vi "Evaluate Alarms.vi"(0 "In Test":bool, 1 "Controller":T1, 2 "Alarm Config":T3, 3 "Data":dbl[](array[numeric]), 4 "Pumps Present":bool[](array[boolean])=[FALSE, FALSE, FALSE, FALSE, FALSE, FALSE], 5 "Trip Counter":i32[](array[numeric]), 6 "Previous Times":u32[](array[numeric]), 7 "Manual CMDs":dbl[](array[numeric]), 9 "Prev ON Times":u32[](array[numeric])) -> (20 "Trip Counter OUT":i32[](array[numeric]), 21 "Previous Times OUT":u32[](array[numeric]), 22 "Alarm Tripped":bool, 24 "Prev ON Times OUT":u32[](array[numeric]), 25 "Alarm Message 1":string, 26 "Alarm Message 2":string)   [LabVIEW 2019]
uses:
  Controls/Alarm Config.ctl
  Controls/Alarm Definition.ctl
  Controls/Alarm Profile Config.ctl
  Controls/Controller Config.ctl
  Type Defs/Controller Names.ctl
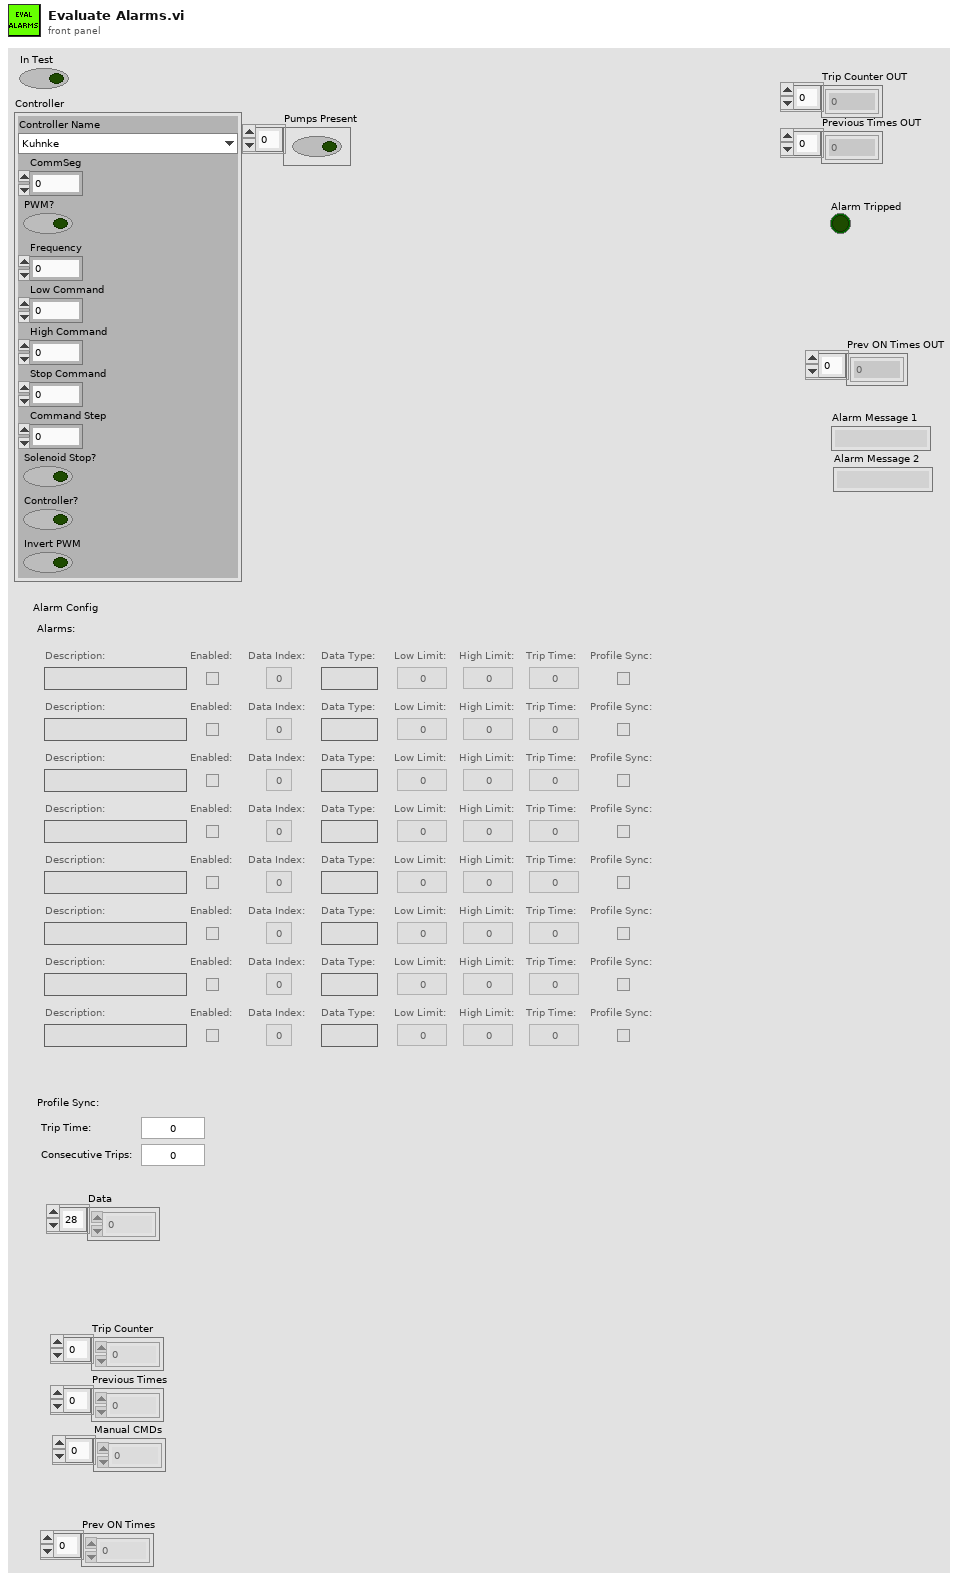
[diagram p1: front panel]
types:
  T1 = typedef "Controller Config.ctl" = cluster{"Controller Name":T2, "CommSeg":i32, "PWM?":bool, "Frequency":i32, "Low Command":dbl, "High Command":dbl, "Stop Command":dbl, "Command Step":dbl, "Solenoid Stop?":bool, "Controller?":bool, "Invert PWM":bool}
  T2 = typedef "Controller Names.ctl" = enum16{"Kuhnke", "Helbako BLDC", "Conti", "Hella BLDC OL PWM", "Hella BLDC Turbine OL PWM", "Hella BLDC Pressure", "Helbako (old)", "TI PWM", "PSA", "Hella Gas", "Hella Diesel", "8 Comm", "10 Comm", "8 Comm Hella", "10 Comm Hella", "8 Comm Omron", "10 Comm Omron", "8 Comm Nissan", "10 Comm Nissan"}
  T3 = typedef "Alarm Config.ctl" = cluster{"Alarms:":T4[], "Profile Sync:":T5}
  T4 = typedef "Alarm Definition.ctl" = cluster{"Description:":string, "Enabled:":bool, "Data Index:":i32, "Data Type:":string, "Low Limit:":dbl, "High Limit:":dbl, "Trip Time:":u32, "Profile Sync:":bool}
  T5 = typedef "Alarm Profile Config.ctl" = cluster{"Trip Time:":u32, "Consecutive Trips:":i32}
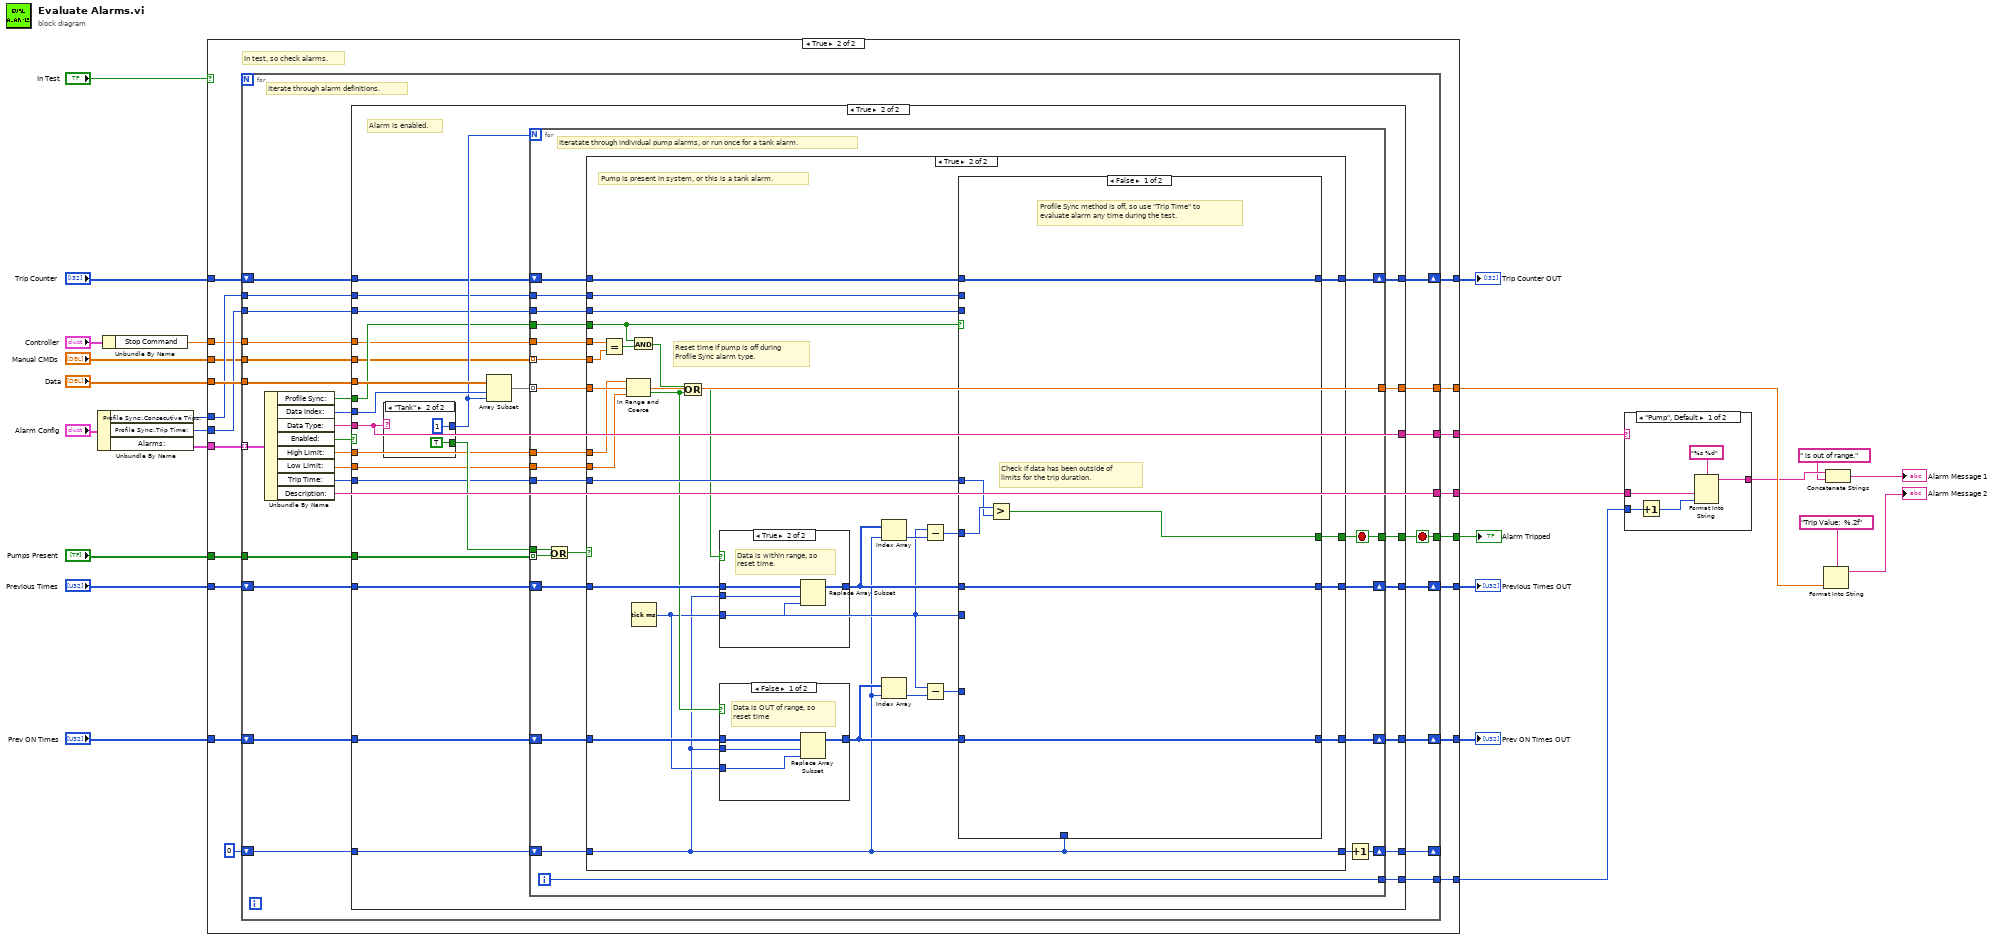
[diagram p0: block diagram]
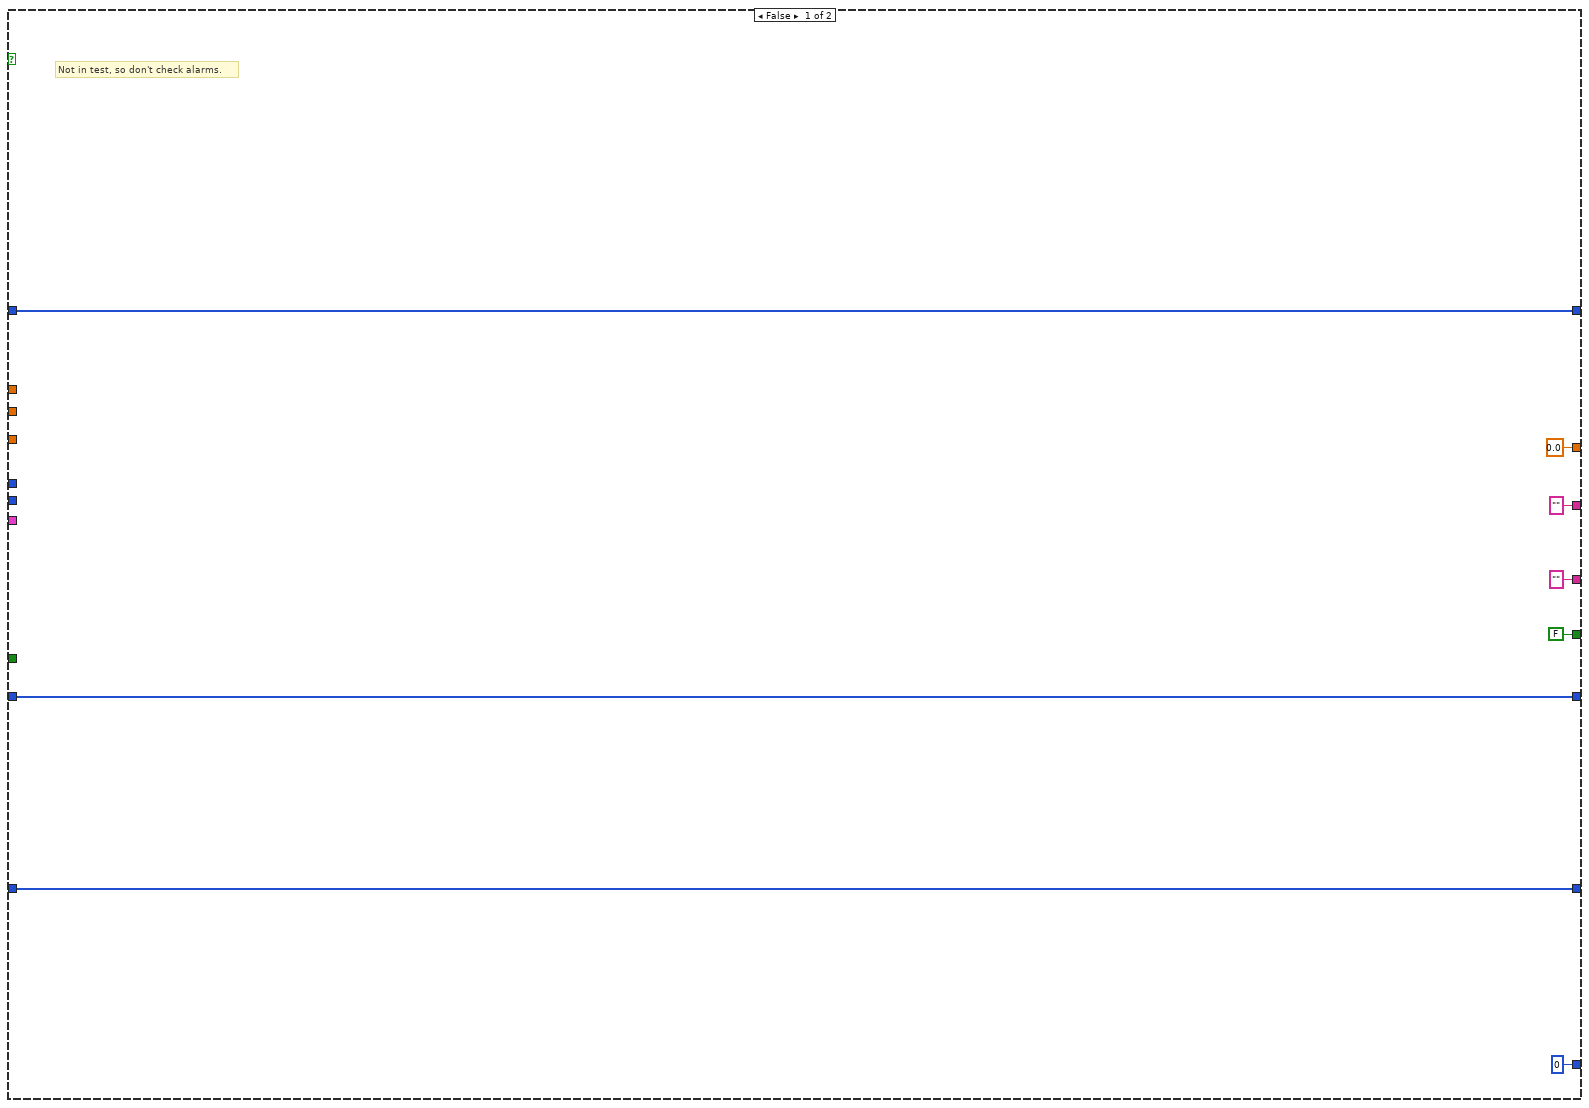
[diagram p3: hidden frame]
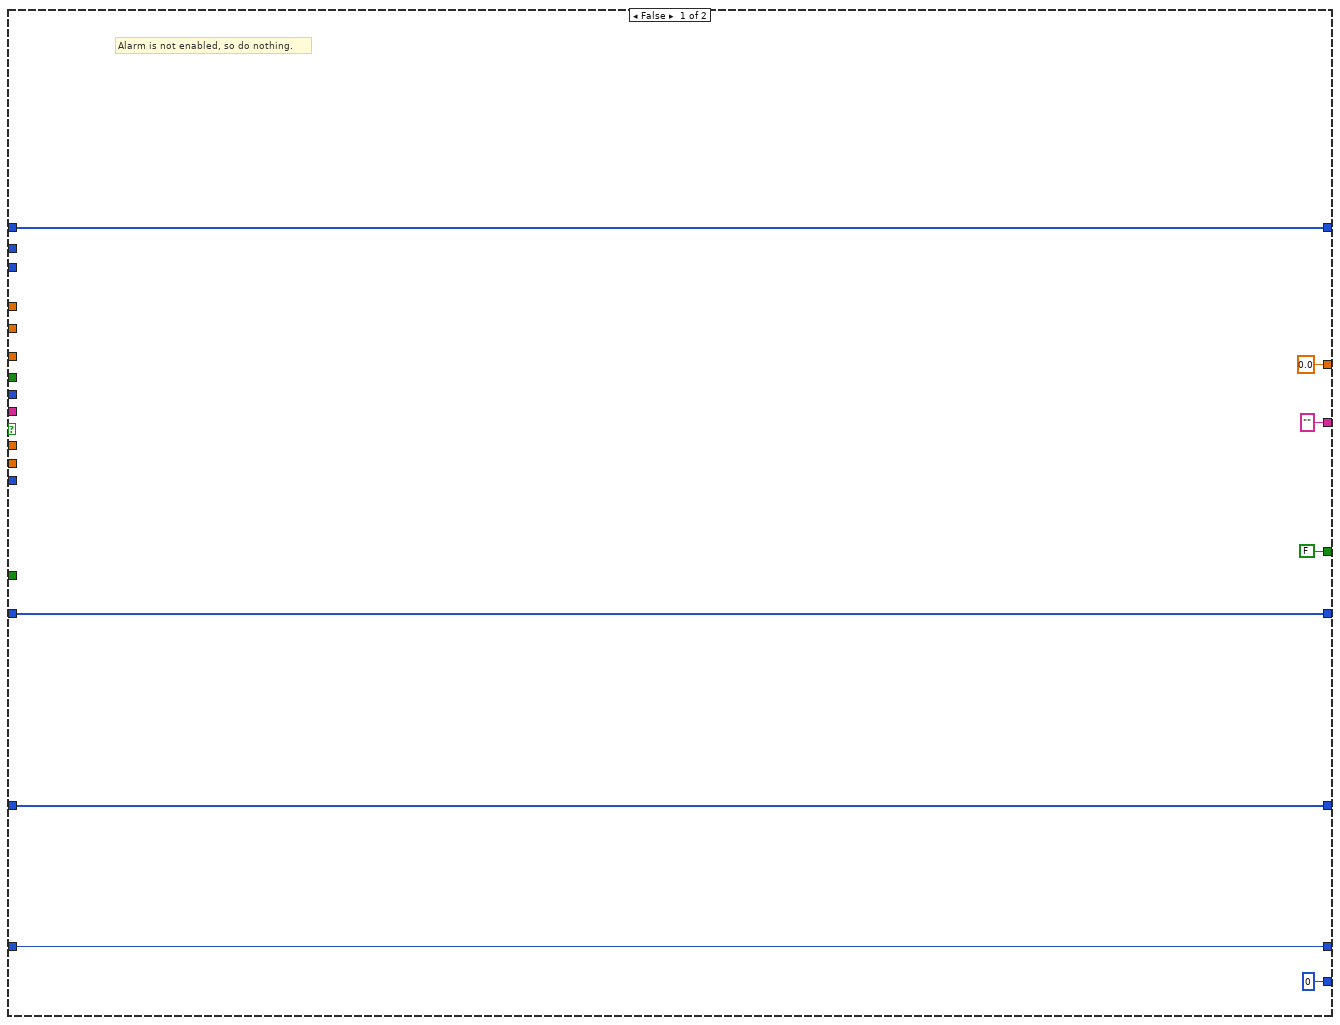
[diagram p4: hidden frame]
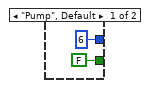
[diagram p5: hidden frame]
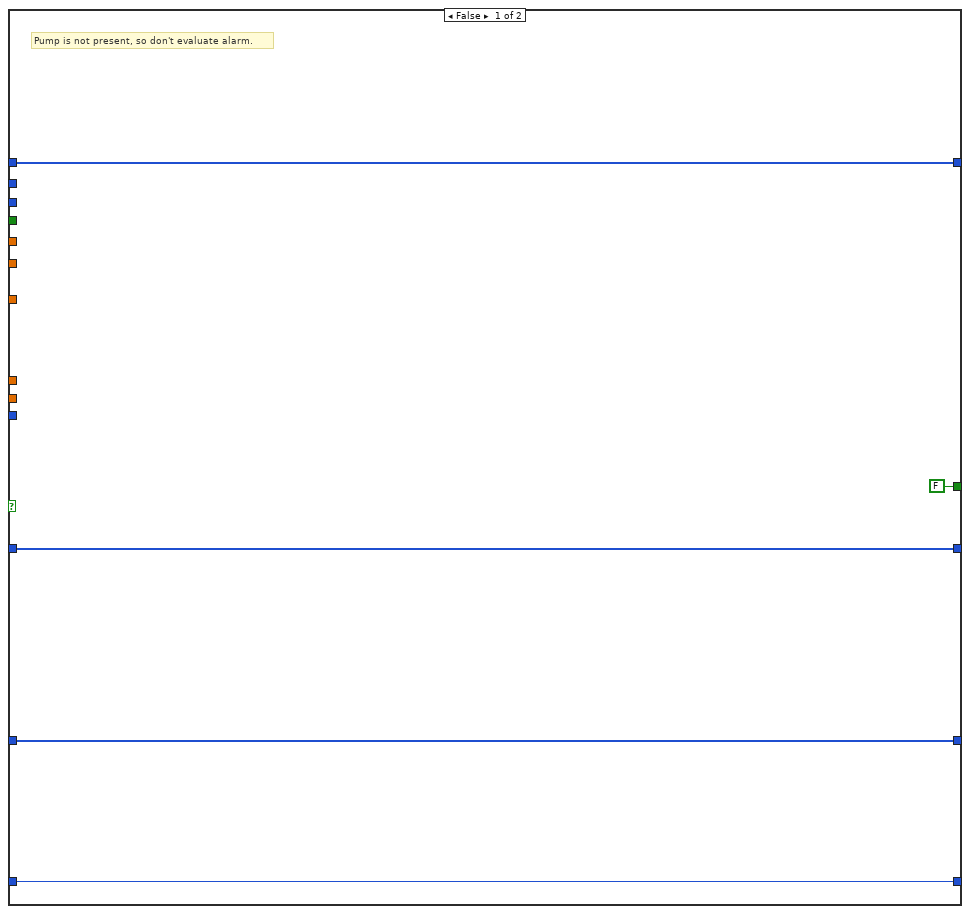
[diagram p6: hidden frame]
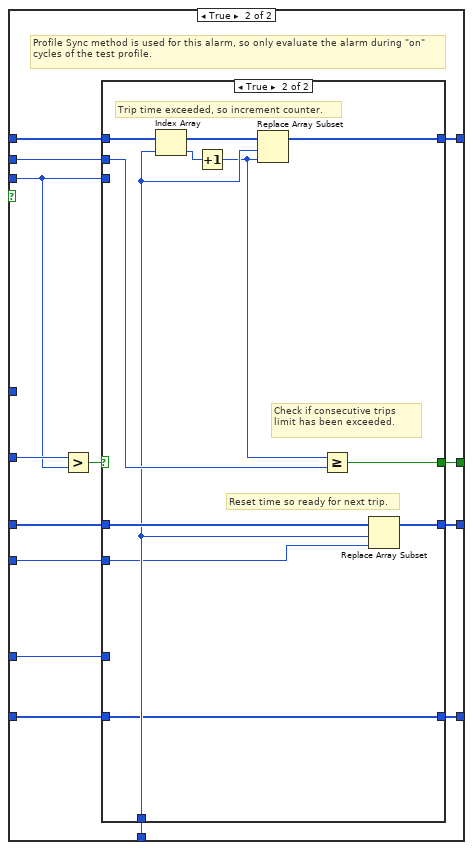
[diagram p9: hidden frame]
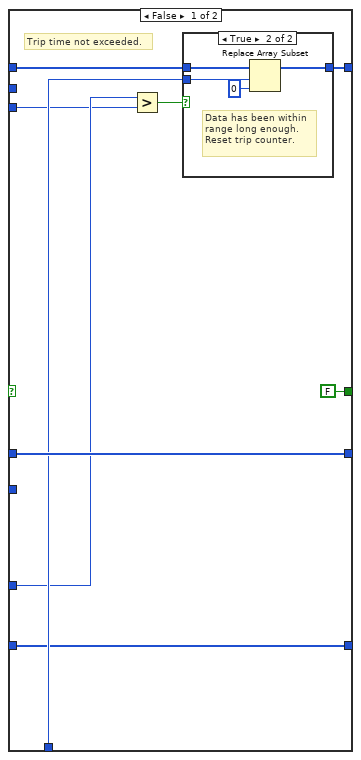
[diagram p10: hidden frame]
diagram:
  n1 = Unbundle By Name("Alarm Config") -> ("Profile Sync:.Consecutive Trips:"=w20:i32, "Profile Sync:.Trip Time:"=w19:u32, "Alarms:"=w23:T4[])
  n2 = Unbundle By Name("Controller") -> ("Stop Command"=w18:dbl)
  n3 = case shown="True" "In Test" {
    tunnel: w23 -> [_ w53]
    tunnel: "Data" -> [_ w52]
    tunnel: "Pumps Present" -> [_ w51]
    tunnel: "Previous Times" -> [w33 w50]
    tunnel: "Trip Counter" -> [w34 w48]
    tunnel: w20 -> [_ w47]
    tunnel: w19 -> [_ w46]
    tunnel: w18 -> [_ w45]
    tunnel: "Manual CMDs" -> [_ w44]
    tunnel: [w34 w43] -> w15
    tunnel: [w33 w42] -> w14
    tunnel: [FALSE w41] -> w13
    tunnel: ["" ("Description:") w40] -> w11
    tunnel: [0 w39] -> w10
    tunnel: ["" ("Data Type:") w38] -> w12
    tunnel: [0.0 w37] -> w6
    tunnel: "Prev ON Times" -> [w27 w36]
    tunnel: [w27 w35] -> w8
    frame False {
      # "Not in test, so don't check alarms."
    }
    frame True {
      # "In test, so check alarms."
      n4 = for {
        tunnel: w53 -> [w80] mode=indexing
        tunnel: w52 -> [w78]
        tunnel: w51 -> [w75]
        shift-right: [w70] -> w42
        shift-left: w50 -> [w71]
        shift-right: [w67] -> _
        shift-left: 0 ("index") -> [w68]
        shift-right: [w65] -> w43
        shift-left: w48 -> [w66]
        tunnel: w47 -> [w64]
        tunnel: w46 -> [w63]
        tunnel: w45 -> [w62]
        tunnel: w44 -> [w61]
        tunnel: [w60] -> w41
        tunnel: [w59] -> w40
        tunnel: [w58] -> w39
        tunnel: [w57] -> w38
        tunnel: [w56] -> w37
        shift-right: [w54] -> w35
        shift-left: w36 -> [w55]
        stop <- w60 stop-if-true
        # "Iterate through alarm definitions."
        n5 = Unbundle By Name(w80) -> ("Profile Sync:"=w69:bool, "Data Index:"=w77:i32, "Data Type:"=w76:string, "Enabled:"=w79:bool, "High Limit:"=w74:dbl, "Low Limit:"=w73:dbl, "Trip Time:"=w72:u32, "Description:"=w59:string)
        n6 = case shown="True" w79 {
          tunnel: w78 -> [_ w114]
          tunnel: w77 -> [_ w113]
          tunnel: w76 -> [_ w92]
          tunnel: w75 -> [_ w110]
          tunnel: w74 -> [_ w109]
          tunnel: w73 -> [_ w108]
          tunnel: w72 -> [_ w107]
          tunnel: w71 -> [w86 w105]
          tunnel: [w86 w104] -> w70
          tunnel: w69 -> [_ w103]
          tunnel: w68 -> [w85 w102]
          tunnel: [w85 w101] -> w67
          tunnel: [FALSE w100] -> w60
          tunnel: w66 -> [w88 w99]
          tunnel: [w88 w98] -> w65
          tunnel: w64 -> [_ w97]
          tunnel: w63 -> [_ w96]
          tunnel: w62 -> [_ w95]
          tunnel: w61 -> [_ w94]
          tunnel: [0 w93] -> w58
          tunnel: ["" ("Data Type:") w92] -> w57
          tunnel: [0.0 w91] -> w56
          tunnel: w55 -> [w81 w90]
          tunnel: [w81 w89] -> w54
          frame False {
            # "Alarm is not enabled, so do nothing."
          }
          frame True {
            # "Alarm is enabled."
            n7 = case shown="\"Tank\"" w92 {
              tunnel: [6 ("length") 1 ("length")] -> w112
              tunnel: [FALSE TRUE] -> w111
              frame "Pump", Default {
              }
              frame "Tank" {
              }
            }
            n8 = Array Subset(array=w114, index=w113, length=w112) -> (w106:dbl[])
            n9 = for {
              N: w112 -> [_]
              tunnel: w111 -> [w141]
              tunnel: w110 -> [w140] mode=indexing
              tunnel: w109 -> [w138]
              tunnel: w108 -> [w137]
              tunnel: w107 -> [w136]
              tunnel: w106 -> [w122] mode=indexing
              shift-right: [w134] -> w104
              shift-left: w105 -> [w135]
              tunnel: w103 -> [w133]
              shift-right: [w123] -> w101
              shift-left: w102 -> [w132]
              tunnel: [w131] -> w100
              shift-right: [w129] -> w98
              shift-left: w99 -> [w130]
              tunnel: w97 -> [w128]
              tunnel: w96 -> [w127]
              tunnel: w95 -> [w126]
              tunnel: w94 -> [w125] mode=indexing
              tunnel: [w119] -> w93
              tunnel: [w122] -> w91
              shift-right: [w120] -> w89
              shift-left: w90 -> [w121]
              i -> [w119]
              stop <- w131 stop-if-true
              # "Iteratate through individual pump alarms, or run once for a tank alarm."
              n10 = Or(x=w141, y=w140) -> (x .or. y?=w139:bool)
              n11 = case shown="True" w139 {
                tunnel: w138 -> [_ w174]
                tunnel: w137 -> [_ w173]
                tunnel: w136 -> [_ w169]
                tunnel: w122 -> [_ w148]
                tunnel: w135 -> [w144 w172]
                tunnel: [w144 w157] -> w134
                tunnel: w133 -> [_ w161]
                tunnel: w132 -> [w143 w147]
                tunnel: [w143 w147] -> w124
                tunnel: [FALSE w170] -> w131
                tunnel: w130 -> [w146 w168]
                tunnel: [w146 w167] -> w129
                tunnel: w128 -> [_ w166]
                tunnel: w127 -> [_ w165]
                tunnel: w126 -> [_ w164]
                tunnel: w125 -> [_ w163]
                tunnel: w121 -> [w142 w155]
                tunnel: [w142 w152] -> w120
                frame False {
                  # "Pump is not present, so don't evaluate alarm."
                }
                frame True {
                  # "Reset time if pump is off during\nProfile Sync alarm type."
                  # "Pump is present in system, or this is a tank alarm."
                  n12 = Equal?(x=w164, y=w163) -> (x = y?=w162:bool)
                  n13 = In Range and Coerce(upper limit=w174, x=w148, lower limit=w173) -> (In Range?=w156:bool)  [unwired: 1 out]
                  n14 = And(x=w161, y=w162) -> (x .and. y?=w160:bool)
                  n15 = Tick Count (ms)() -> (millisecond timer value=w153:u32)
                  n16 = Or(x=w160, y=w156) -> (x .or. y?=w159:bool)
                  n17 = case shown="True" w159 {
                    tunnel: w172 -> [w180 w184]
                    tunnel: [w180 w183] -> w158
                    tunnel: w147 -> [_ w182]
                    tunnel: w153 -> [_ w181]
                    frame False {
                      # "Data is out of range, so\nmaintain previous time."
                    }
                    frame True {
                      # "Data is within range, so\nreset time."
                      n18 = Replace Array Subset(array=w184, new element=w181, index=w182) -> (w183:u32[])
                    }
                  }
                  n19 = case shown="False" w156 {
                    tunnel: w155 -> [w178 w179]
                    tunnel: [w177 w179] -> w151
                    tunnel: w147 -> [w176 _]
                    tunnel: w153 -> [w175 _]
                    frame False {
                      # "Data is OUT of range, so\nreset time"
                      n20 = Replace Array Subset(array=w178, new element=w175, index=w176) -> (w177:u32[])
                    }
                    frame True {
                      # "Data is WITHIN range, so\nmaintain previous time."
                    }
                  }
                  n21 = Index Array(array=w158, index=w147) -> (element=w171:u32)
                  n22 = Index Array(array=w151, index=w147) -> (element=w154:u32)
                  n23 = Subtract(x=w153, y=w171) -> (x-y=w150:u32)
                  n24 = Subtract(x=w153, y=w154) -> (x-y=w149:u32)
                  n25 = case shown="False" w161 {
                    tunnel: [w188 w198] -> w170
                    tunnel: w150 -> [w190 w204]
                    tunnel: w169 -> [w189 _]
                    tunnel: w168 -> [w187 w203]
                    tunnel: [w187 w202] -> w167
                    tunnel: w166 -> [_ w199]
                    tunnel: w165 -> [_ w191]
                    tunnel: w147 -> [_ w200]
                    tunnel: w158 -> [w186 w197]
                    tunnel: [w186 w196] -> w157
                    tunnel: w153 -> [_ w195]
                    tunnel: w151 -> [w185 w194]
                    tunnel: [w185 w193] -> w152
                    tunnel: w149 -> [_ w192]
                    frame False {
                      # "Check if data has been outside of\nlimits for the trip duration."
                      # "Profile Sync method is off, so use \"Trip Time\" to\nevaluate alarm any time during the test."
                      n26 = Greater?(x=w190, y=w189) -> (0:w188:bool)
                    }
                    frame True {
                      # "Profile Sync method is used for this alarm, so only evaluate the alarm during \"on\" cycles of the test profile."
                      n27 = Greater?(x=w204, y=w191) -> (0:w201:bool)
                      n28 = case shown="True" w201 {
                        tunnel: [w210 w229] -> w202
                        tunnel: w203 -> [w211 w228]
                        tunnel: w200 -> [w209 w222]
                        tunnel: w199 -> [_ w226]
                        tunnel: [FALSE w225] -> w198
                        tunnel: w197 -> [w212 w224]
                        tunnel: [w212 w223] -> w196
                        tunnel: w195 -> [_ w221]
                        tunnel: [w205 w220] -> w193
                        tunnel: w194 -> [w205 w220]
                        tunnel: w192 -> [w208 _]
                        tunnel: w191 -> [w207 _]
                        frame False {
                          # "Trip time not exceeded."
                          n29 = Greater?(x=w208, y=w207) -> (0:w206:bool)
                          n30 = case shown="True" w206 {
                            tunnel: w211 -> [w214 w218]
                            tunnel: [w214 w217] -> w210
                            tunnel: w209 -> [_ w216]
                            frame False {
                              # "Data has NOT come\ncome back into range\nlong enough.\nMaintain counters."
                            }
                            frame True {
                              # "Data has been within\nrange long enough. \nReset trip counter."
                              n31 = Replace Array Subset(array=w218, new element=0 ("new element/subarray"), index=w216) -> (w217:i32[])
                            }
                          }
                        }
                        frame True {
                          # "Reset time so ready for next trip."
                          # "Check if consecutive trips limit has been exceeded."
                          # "Trip time exceeded, so increment counter."
                          n32 = Index Array(array=w228, index=w222) -> (element=w227:i32)
                          n33 = Increment(x=w227) -> (x+1=w219:i32)
                          n34 = Replace Array Subset(array=w228, new element=w219, index=w222) -> (w229:i32[])
                          n35 = Greater Or Equal?(x=w219, y=w226) -> (x >= y?=w225:bool)
                          n36 = Replace Array Subset(array=w224, new element=w221, index=w222) -> (w223:u32[])
                        }
                      }
                    }
                  }
                }
              }
              n37 = Increment(x=w124) -> (x+1=w123:i32)
            }
          }
        }
      }
    }
  }
  "Trip Counter OUT" <- w15
  "Previous Times OUT" <- w14
  "Alarm Tripped" <- w13
  "Prev ON Times OUT" <- w8
  n38 = case shown="\"Pump\", Default" w12 {
    tunnel: w11 -> [w232 w235]
    tunnel: w10 -> [w231 _]
    tunnel: [w233 w235] -> w3
    frame "Pump", Default {
      n39 = Increment(x=w231) -> (x+1=w230:i32)
      n40 = Format Into String(format string="%s %d", w232, w230) -> (resulting string=w233:string)  [unwired: 2 in, 1 out]
    }
    frame "Tank" {
    }
  }
  n41 = Format Into String(format string="Trip Value:  %.2f", w6) -> (resulting string=→"Alarm Message 2":string)  [unwired: 2 in, 1 out]
  n42 = Concatenate Strings(w3, " is out of range." ("format string")) -> (→"Alarm Message 1":string)
